vi "target menu name.vi"(8 "error in":errorcluster, 11 "PLTarget cRIO in":refnum<class "PLTarget CVS.lvclass">) -> (0 "error out":errorcluster, 2 "menu name":string, 3 "PLTarget cRIO out":refnum<class "PLTarget CVS.lvclass">)   [LabVIEW 2013, in "PLTarget CVS.lvclass"]
uses:
  PLTarget CVS.lvclass
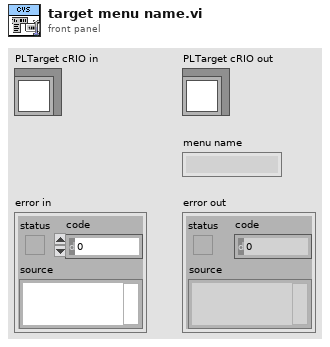
[diagram p1: front panel]
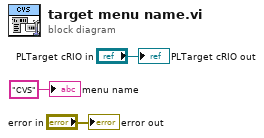
[diagram p0: block diagram]
diagram:
  "error out" <- "error in"
  "PLTarget cRIO out" <- "PLTarget cRIO in"
  "menu name" <- "CVS" ("menu name")
